vi "New.vi"(8 "error in (no error)":errorcluster, 10 "Name":string, 11 "Service in":refnum<class "Service.lvclass">) -> (0 "error out":errorcluster, 3 "Service out":refnum<class "Service.lvclass">)   [LabVIEW 2024, in "Ramses Framework.lvlib" / "Service.lvclass"]
doc: "Instantiates a classes properties, registers with the local server, and stores the server reference into it's local memory."
uses:
  Service.lvclass
  Service.lvclass/Service.ctl
  Communications/Server/Base Server/Server.lvclass
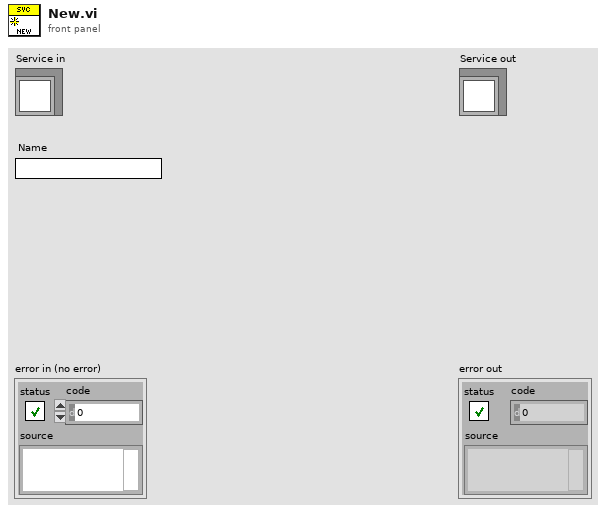
[diagram p1: front panel]
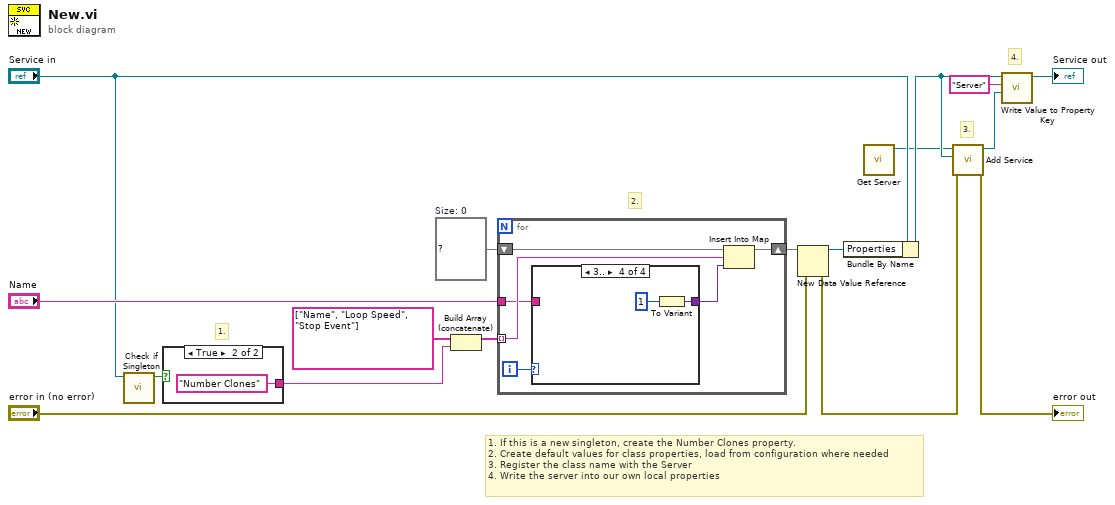
[diagram p0: block diagram]
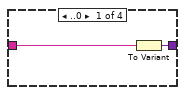
[diagram p3: hidden frame]
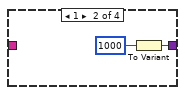
[diagram p4: hidden frame]
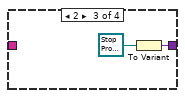
[diagram p5: hidden frame]
diagram:
  w7 = map{string, variant} {}  # Size: 0
  # "4."
  # "3."
  # "2."
  # "1."
  # "1. If this is a new singleton, create the Number Clones property.\n2. Create default values for class properties, load from configuration where needed\n3. Register the class name with the Server\n4. Write the server into our own local properties"
  n1 = call-dynamic "Check if Singleton.vi"("Service in"="Service in") -> ("Singleton?"=w2:bool)  [unwired: 9 in, 1 out]
  n2 = case shown="True" w2 {
    tunnel: [_ "Number Clones" ("String")] -> w4
    frame False {
    }
    frame True {
    }
  }
  n3 = Build Array (concatenate)(string[] ["Name", "Loop Speed", "Stop Event"], w4) -> (w5:string[])
  n4 = for {
    shift-right: [w23] -> w10
    shift-left: w7 -> [w24]
    tunnel: w5 -> [w20] mode=indexing
    tunnel: "Name" -> [w19]
    i -> [w22]
    n5 = case shown="3.." w22 {
      tunnel: [w26 w28 w30 w32] -> w21
      tunnel: w19 -> [w25 _ _ _]
      frame ..0 {
        n6 = To Variant(anything=w25) -> (Variant=w26:variant)
      }
      frame 1 {
        n7 = To Variant(anything=1000) -> (Variant=w28:variant)
      }
      frame 2 {
        n8 = To Variant(anything=refnum<user-event> refnum ("Stop Event")) -> (Variant=w30:variant)
      }
      frame 3.. {
        n9 = To Variant(anything=1) -> (Variant=w32:variant)
      }
    }
    n10 = Insert Into Map(map in=w24, key=w20, value=w21) -> (map out=w23:map{string, variant})  [unwired: 2 out]
  }
  n11 = New Data Value Reference(data value=w10, error in="error in (no error)") -> (data value reference=w14:refnum<data-value>, error out=w12:errorcluster)
  n12 = Bundle By Name(cluster="Service in", "Properties"=w14) -> (w8:refnum<class "Service.lvclass">)
  n13 = call "Get Server.vi"() -> ("Server out"=w1:refnum<class "Server.lvclass">)  [unwired: 10 in, 1 out]
  n14 = call "Add Service.vi"("error in (no error)"=w12, "Service.lvclass"=w8, "Server in"=w1) -> ("error out"=→"error out":errorcluster, "Server out"=w13:refnum<class "Server.lvclass">)  [unwired: 7 in]
  n15 = call "Write Value to Property Key.vi"("Value"=w13, "Key"="Server", "Service in"=w8) -> ("Service out"=→"Service out":refnum<class "Service.lvclass">)  [unwired: 7 in, 1 out]
